vi "DoRefocus.vi"(6 "parameters_z-scan":T2={"dwell_time_ms"=2.0, "q_steps"=5, "span_um"=1.0, "refocus"=TRUE}, 8 "parameters_xy-scan":T3={"image_size_xy_um"=2.0, "frame_size_xy_px"=7, "dwell_time_ms"=0.5}, 9 "time_const":timestamp[](array[timestamp]), 10 "mini_scan":dbl[][][](array[numeric]), 11 "input_xyz":cluster{"X_um":sgl, "Y_um":sgl, "Z_um":sgl}) -> (0 "time_const":timestamp, 1 "mini_scan_all":dbl[][][](array[numeric]), 2 "output_xyz":T1, 4 "time_const_all":timestamp[](array[timestamp]))   [LabVIEW 2018]
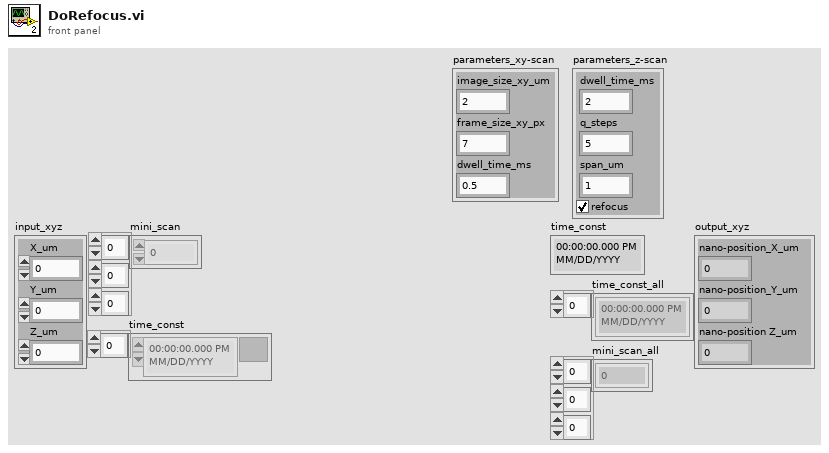
[diagram p1: front panel]
types:
  T1 = cluster{"nano-position_X_um":sgl, "nano-position_Y_um":sgl, "nano-position Z_um":sgl}
  T2 = cluster{"dwell_time_ms":dbl, "q_steps":u32, "span_um":dbl, "refocus":bool}
  T3 = cluster{"image_size_xy_um":dbl, "frame_size_xy_px":u32, "dwell_time_ms":dbl}
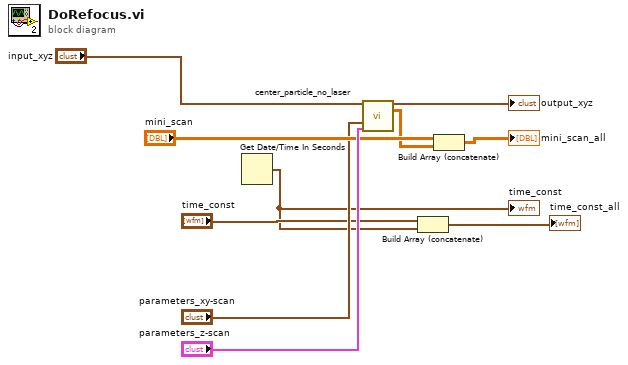
[diagram p0: block diagram]
diagram:
  n1 = Get Date/Time In Seconds() -> (seconds since 1Jan1904=w5:timestamp)
  "time_const" <- w5
  n2 = call "center_particle_no_laser.vi"("input_xyz"="input_xyz", "parameters_xy-scan"="parameters_xy-scan", "parameters_z-scan"="parameters_z-scan") -> ("output_xyz"=→"output_xyz":T1, "mini_scan"=w1:dbl[][])  [unwired: 11 in]
  n3 = Build Array (concatenate)("time_const", w5) -> (→"time_const_all":timestamp[])
  n4 = Build Array (concatenate)("mini_scan", w1) -> (→"mini_scan_all":dbl[][][])
